vi "圆环到矩形转换.vi"(9 "Radius":dbl, 10 "CenerY":dbl, 11 "CenerX":dbl) -> (3 "Bounding Rectangle out":T1)   [LabVIEW 2017]
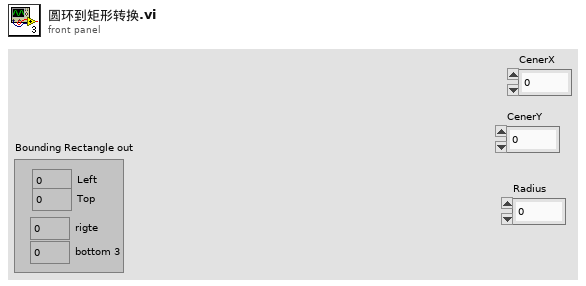
[diagram p1: front panel]
types:
  T1 = cluster{"Left":i32, "Top":i32, "rigte":i32, "bottom 3":i32}
  T2 = cluster{"Left":i32, "Top":i32, "Right":i32, "Bottom":i32}
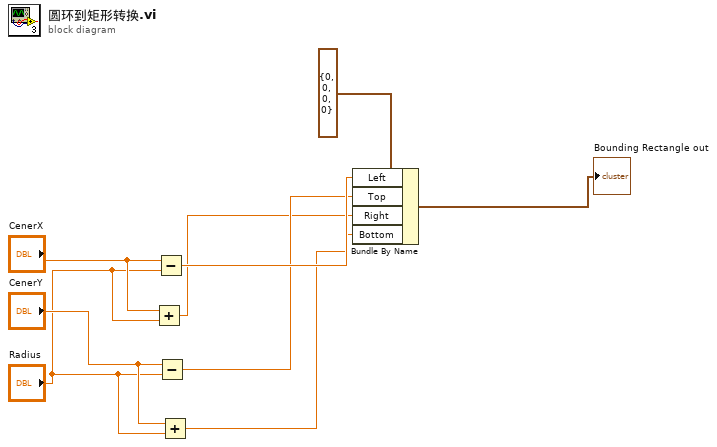
[diagram p0: block diagram]
diagram:
  n1 = Add(x="CenerX", y="Radius") -> (x+y=w4:dbl)
  n2 = Subtract(x="CenerX", y="Radius") -> (x-y=w7:dbl)
  n3 = Subtract(x="CenerY", y="Radius") -> (x-y=w6:dbl)
  n4 = Add(x="CenerY", y="Radius") -> (x+y=w1:dbl)
  n5 = Bundle By Name(cluster=T2 {"Left"=0, "Top"=0, "Right"=0, "Bottom"=0} ("Bounding Rectangle out 2"), "Left"=w7, "Top"=w6, "Right"=w4, "Bottom"=w1) -> (→"Bounding Rectangle out":T2)
